vi "example cycle thijs.vi"() -> ()   [LabVIEW 2016]
panel:
  in  "position y":i32
  in  "position x":i32
  in  "revolution 2":i32
  in  "angle 2":u32
  out "revolution":i32
  out "angle":u32
  out "pos y":i32
  out "pos x":i32
  in  "Frequency rotation":u32=8000 min=1 max=18500 step=1
  in  "Amplitude rotation":u32=4000 min=1 max=4000 step=1
  in  "Steps rotation":i32=1000 min=0 max=1000000 step=1
  in  "System Locator":string="usb:ix:0"
  in  "Numeric":i32=1
  out "Error":errorcluster
  in  "Steps":i32=1000 max=1000000 step=1
  in  "Amplitude":u32=4000 min=1 max=4000 step=1
  in  "Frequency":u32=8000 min=1 max=18500 step=1
  in  "Rotation channel":u32
  in  "Y channel":u32=2
  in  "X channel":u32=1
  out "System Index":u32
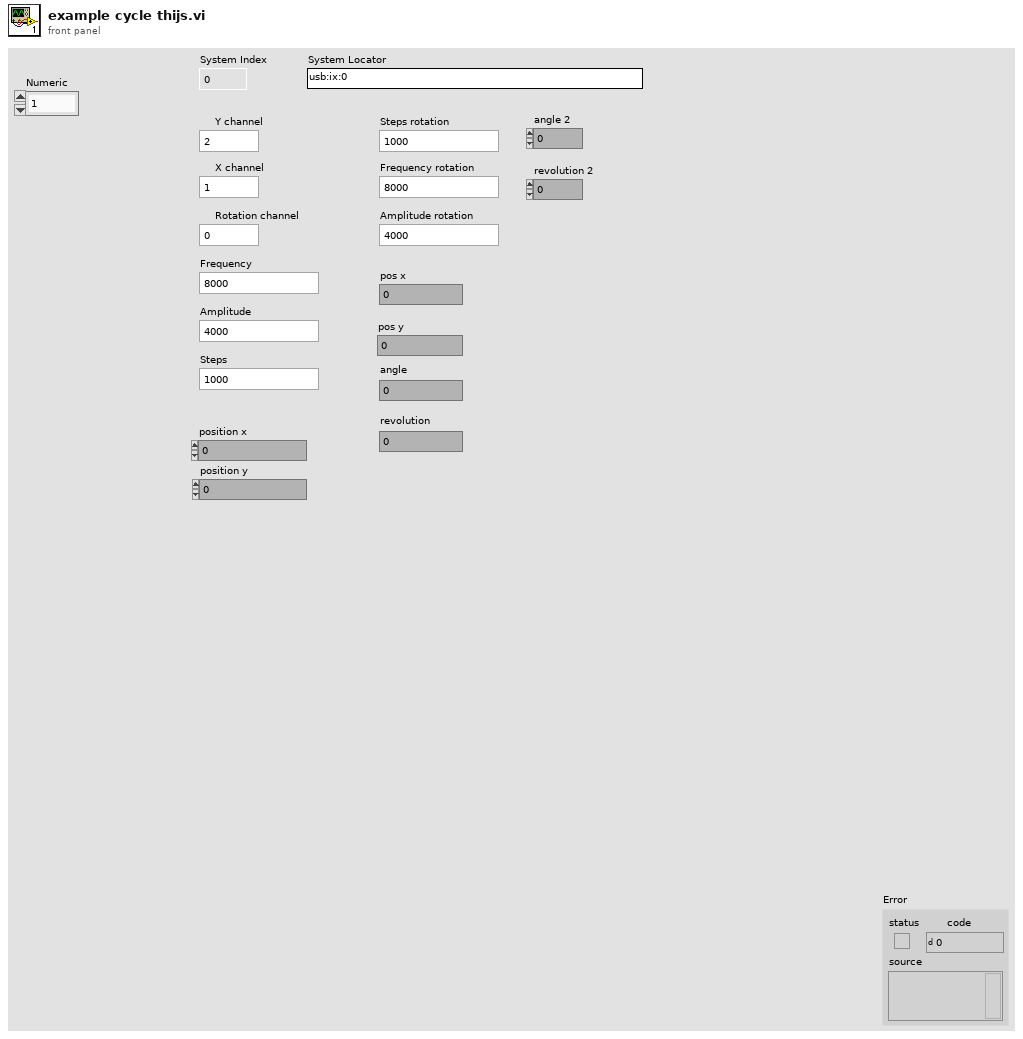
[diagram p1: front panel]
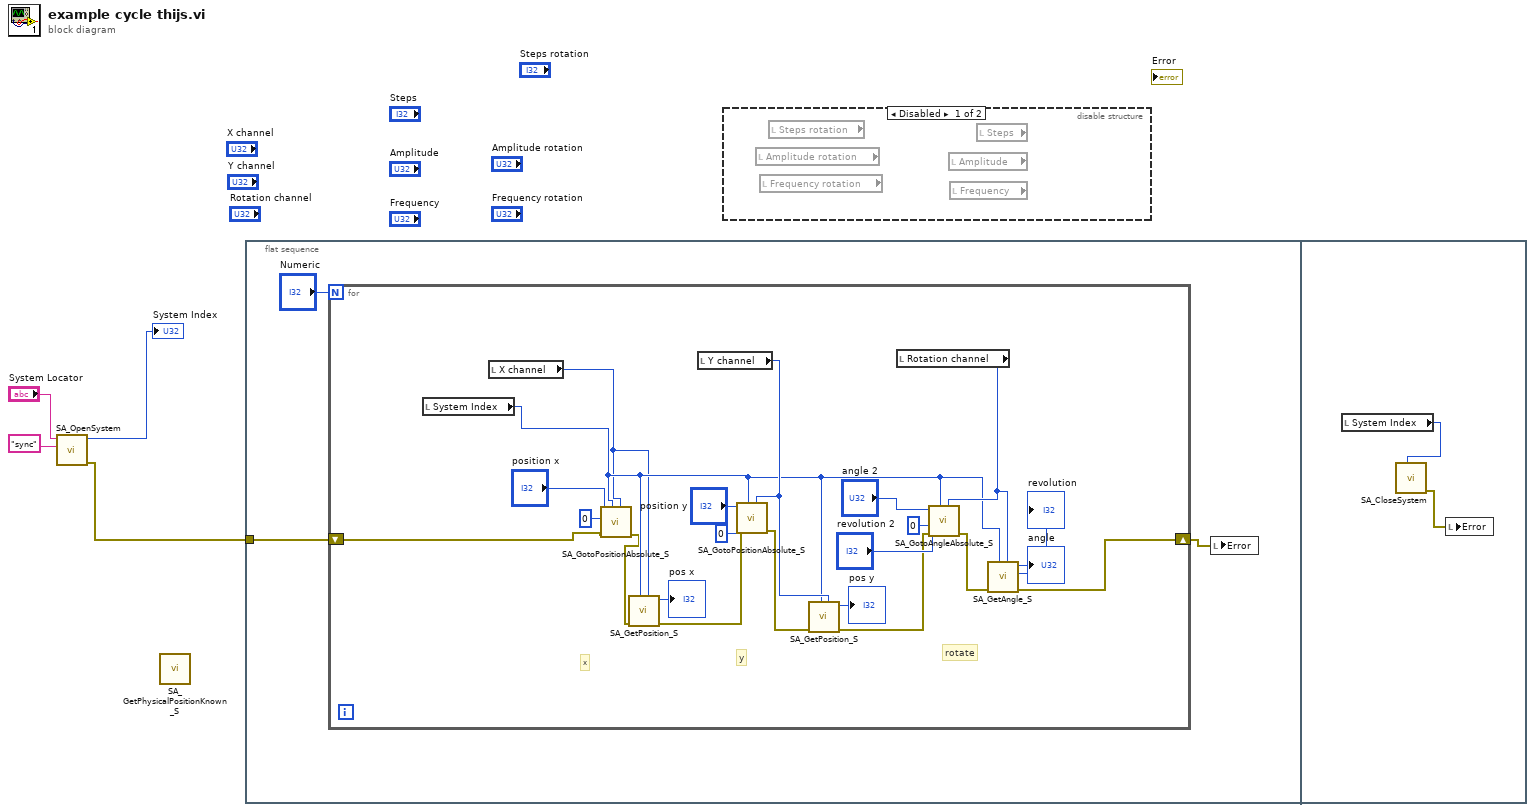
[diagram p0: block diagram]
diagram:
  n1 = call <vilib>:"SA_OpenSystem.vi"("options"="sync", "systemLocator"="System Locator") -> ("error out"=w1:errorcluster, "systemIndexOut"=→"System Index":u32)  [unwired: 8 in]
  n2 = call <vilib>:"SA_GetPhysicalPositionKnown_S.vi"() -> ()  [unwired: 10 in, 2 out]
  n3 = flat-sequence {
    tunnel: w1 -> [w6]
    frame #0 {
      n4 = for {
        N: "Numeric" -> [_]
        shift-right: [w22] -> w5
        shift-left: w6 -> [w12]
        # "rotate"
        # "y"
        # "x"
        n5 = local read "System Index"() -> (w15:u32)
        n6 = local read "X channel"() -> (w14:u32)
        n7 = call <vilib>:"SA_GotoPositionAbsolute_S.vi"("channelIndex"=w14, "systemIndex"=w15, "error in (no error)"=w12, "holdTime"=u32 0, "position"="position x") -> ("error out"=w13:errorcluster)  [unwired: 6 in]
        n8 = call <vilib>:"SA_GetPosition_S.vi"("channelIndex"=w14, "systemIndex"=w15, "error in (no error)"=w13) -> ("error out"=w29:errorcluster, "position"=→"pos x":i32)  [unwired: 7 in]
        n9 = local read "Y channel"() -> (w26:u32)
        n10 = call <vilib>:"SA_GotoPositionAbsolute_S.vi"("channelIndex"=w26, "systemIndex"=w15, "error in (no error)"=w29, "holdTime"=u32 0, "position"="position y") -> ("error out"=w25:errorcluster)  [unwired: 6 in]
        n11 = call <vilib>:"SA_GetPosition_S.vi"("channelIndex"=w26, "systemIndex"=w15, "error in (no error)"=w25) -> ("error out"=w17:errorcluster, "position"=→"pos y":i32)  [unwired: 7 in]
        n12 = local read "Rotation channel"() -> (w21:u32)
        n13 = call <vilib>:"SA_GotoAngleAbsolute_S.vi"("channelIndex"=w21, "systemIndex"=w15, "error in (no error)"=w17, "holdTime"=u32 0, "revolution"="revolution 2", "angle"="angle 2") -> ("error out"=w20:errorcluster)  [unwired: 5 in]
        n14 = call <vilib>:"SA_GetAngle_S.vi"("channelIndex"=w21, "systemIndex"=w15, "error in (no error)"=w20) -> ("error out"=w22:errorcluster, "revolution"=→"revolution":i32, "angle"=→"angle":u32)  [unwired: 6 in]
      }
      n15 = local write "Error"(w5) -> ()
    }
    frame #1 {
      n16 = local read "System Index"() -> (w31:u32)
      n17 = call <vilib>:"SA_CloseSystem.vi"("systemIndex"=w31) -> ("error out"=w30:errorcluster)  [unwired: 10 in]
      n18 = local write "Error"(w30) -> ()
    }
  }
  n19 = disable-structure shown="Disabled" {
    frame Disabled {
      n20 = local read "Amplitude rotation"() -> ()  [unwired: 1 out]
      n21 = local read "Frequency rotation"() -> ()  [unwired: 1 out]
      n22 = local read "Steps rotation"() -> ()  [unwired: 1 out]
      n23 = local read "Amplitude"() -> ()  [unwired: 1 out]
      n24 = local read "Frequency"() -> ()  [unwired: 1 out]
      n25 = local read "Steps"() -> ()  [unwired: 1 out]
    }
    frame Enabled {
    }
  }
